vi "Steppers_and_Scanners_control_6_15.vi"(1 "ANC300 address":refnum<visa-resource-name>="COM8") -> (18 "Serial":string="ANC300B-C-2133-4009033")   [LabVIEW 2024]
panel:
  in  "wait time (ms)":u32=300
  out "2: Voltage Reading":dbl format="%#_13g"
  out "1: Voltage Reading":dbl format="%#_13g"
  in  "Set/Read":bool=TRUE
  in  "Stepper 4":bool
  in  "4: number of steps":i32=1
  in  "4: stepping direction":bool=TRUE
  in  "4: AC Voltage":dbl=60.0 min=0.0 format="%.1f"
  in  "4: AC frequency":dbl=300.0 min=0.0 format="%.1f"
  in  "Stepper 3":bool
  in  "3: number of steps":i32=1
  in  "3: stepping direction":bool=TRUE
  in  "3: AC Voltage":dbl=60.0 min=0.0 format="%.1f"
  in  "3: AC frequency":dbl=300.0 min=0.0 format="%.1f"
  in  "2: ms to wait":u32=30
  in  "2: Offset Voltage":dbl min=0.0 format="%.2g"
  in  "1: ms to wait":u32=30
  in  "1: Offset Voltage":dbl min=0.0 format="%.2f"
  # "scanner limits: 150V at 2K. 60V at 300K"
  # "Scanner 1"
  # "Scanner 2"
  # "59"
  # "66"
  # "1. Shouldn't have to change the ms to wait times. \n2. If the piezos aren't moving, it's probably because they need to be exercised first. Best to do that manually\nwith the switches on the board or by moving it here several steps at a time with a high AC voltage. If it doesn't move, you have to rerun the file because it is waiting for it to move and will get stuck there if it isn't moving.\n3. Set 'low temperature' or 'high temperature' limits on the controller manually. You can't do that remotely.  DONT GO ABOVE 60V"
  # "Move Stepper 3 Once"
  # "Move Stepper 4 Once"
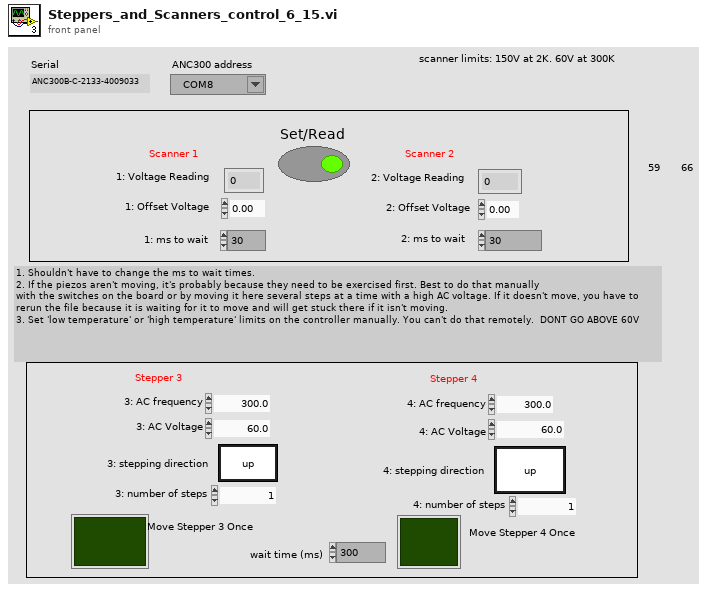
[diagram p1: front panel]
types:
  T1 = cluster{"error ":bool, "error number":i32, "error code":string}
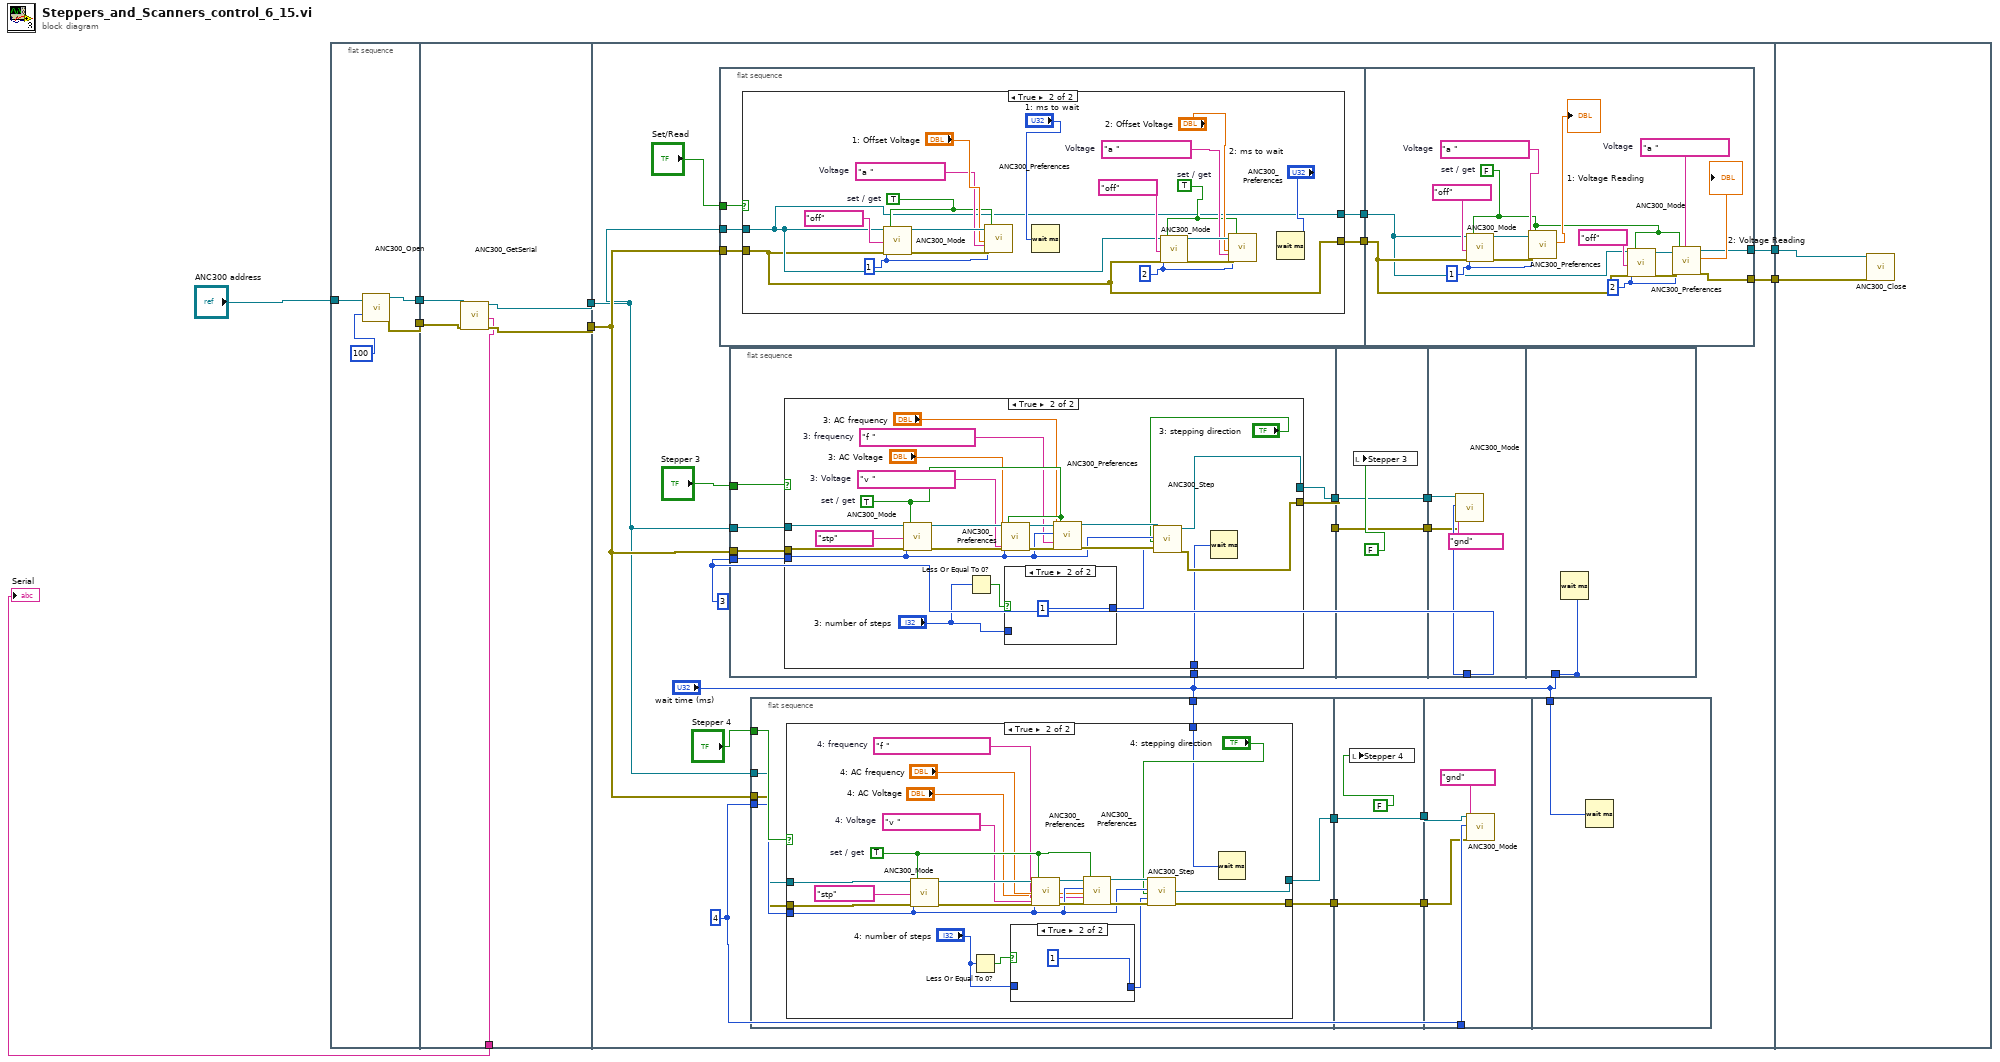
[diagram p0: block diagram]
diagram:
  n1 = flat-sequence {
    tunnel: "ANC300 address" -> [w11]
    tunnel: [w12] -> w8
    tunnel: [w10] -> w7
    tunnel: w8 -> [w17]
    tunnel: w7 -> [w16]
    tunnel: [w15] -> w6
    tunnel: [w14] -> w5
    tunnel: [w13] -> w4
    tunnel: w6 -> [w34]
    tunnel: w5 -> [w35]
    tunnel: [w19] -> w2
    tunnel: [w18] -> w1
    tunnel: w2 -> [w163]
    tunnel: w1 -> [w162]
    frame #0 {
      n2 = call "ANC300_Open.vi"("ANC300 Communication Port In"=w11, "milliseconds to wait"=u32 100 ("millisecond timer value")) -> ("ANC300 Communication Port Out"=w12:refnum<visa-resource-name>, "error out"=w10:T1)  [unwired: 13 in, 3 out]
    }
    frame #1 {
      n3 = call "ANC300_GetSerial.vi"("ANC300 Communication Port In"=w17, "error in"=w16) -> ("ANC300 Communication Port Out"=w15:refnum<visa-resource-name>, "Serial"=w13:string, "error out"=w14:T1)  [unwired: 10 in, 5 out]
    }
    frame #2 {
      w33 = 3
      w36 = 4
      n4 = flat-sequence {
        tunnel: w35 -> [w42]
        tunnel: w34 -> [w41]
        tunnel: "Set/Read" -> [w40]
        tunnel: [w39] -> w26
        tunnel: [w38] -> w25
        tunnel: w26 -> [w68]
        tunnel: w25 -> [w69]
        tunnel: [w64] -> w19
        tunnel: [w63] -> w18
        frame #0 {
          n5 = case shown="True" w40 {
            tunnel: w42 -> [w43 w45]
            tunnel: w41 -> [w44 w46]
            tunnel: [w44 w46] -> w39
            tunnel: [w43 w45] -> w38
            frame False {
            }
            frame True {
              w47 = 2
              w48 = 1
              w49 = TRUE  # set / get
              w52 = "a "  # Voltage
              w56 = TRUE  # set / get
              w59 = "a "  # Voltage
              n6 = call "ANC300_Mode.vi"("ANC300 Communication Port In"=w46, "Axis"=w48, "axis mode in"="off", "error in"=w45, "set / get"=w56) -> ("ANC300 Communication Port Out"=w62:refnum<visa-resource-name>, "error out"=w61:T1)  [unwired: 8 in, 5 out]
              n7 = call "ANC300_Preferences.vi"("ANC300 Communication Port In"=w62, "Axis"=w48, "value in"="1: Offset Voltage", "parameter"=w59, "error in"=w61, "set / get"=w56) -> ()  [unwired: 6 in, 8 out]
              n8 = Wait (ms)(milliseconds to wait="1: ms to wait") -> ()  [unwired: 1 out]
              n9 = call "ANC300_Mode.vi"("ANC300 Communication Port In"=w46, "Axis"=w47, "axis mode in"="off", "error in"=w45, "set / get"=w49) -> ("ANC300 Communication Port Out"=w55:refnum<visa-resource-name>, "error out"=w54:T1)  [unwired: 8 in, 5 out]
              n10 = call "ANC300_Preferences.vi"("ANC300 Communication Port In"=w55, "Axis"=w47, "value in"="2: Offset Voltage", "parameter"=w52, "error in"=w54, "set / get"=w49) -> ()  [unwired: 6 in, 8 out]
              n11 = Wait (ms)(milliseconds to wait="2: ms to wait") -> ()  [unwired: 1 out]
            }
          }
        }
        frame #1 {
          w70 = 2
          w71 = 1
          w73 = "a "  # Voltage
          w65 = FALSE  # set / get
          w77 = "a "  # Voltage
          n12 = call "ANC300_Mode.vi"("ANC300 Communication Port In"=w68, "Axis"=w71, "axis mode in"="off", "error in"=w69, "set / get"=w65) -> ("ANC300 Communication Port Out"=w79:refnum<visa-resource-name>, "error out"=w78:T1)  [unwired: 8 in, 5 out]
          n13 = call "ANC300_Preferences.vi"("ANC300 Communication Port In"=w79, "Axis"=w71, "parameter"=w77, "error in"=w78, "set / get"=w65) -> ("value out"=→"1: Voltage Reading":dbl)  [unwired: 7 in, 7 out]
          n14 = call "ANC300_Mode.vi"("ANC300 Communication Port In"=w68, "Axis"=w70, "axis mode in"="off", "error in"=w69, "set / get"=w65) -> ("ANC300 Communication Port Out"=w75:refnum<visa-resource-name>, "error out"=w74:T1)  [unwired: 8 in, 5 out]
          n15 = call "ANC300_Preferences.vi"("ANC300 Communication Port In"=w75, "Axis"=w70, "parameter"=w73, "error in"=w74, "set / get"=w65) -> ("ANC300 Communication Port Out"=w64:refnum<visa-resource-name>, "value out"=→"2: Voltage Reading":dbl, "error out"=w63:T1)  [unwired: 7 in, 5 out]
        }
      }
      n16 = flat-sequence {
        tunnel: "Stepper 3" -> [w86]
        tunnel: w33 -> [w85]
        tunnel: w34 -> [w84]
        tunnel: w35 -> [w83]
        tunnel: [w82] -> w28
        tunnel: [w81] -> w23
        tunnel: "wait time (ms)" -> [w80]
        tunnel: [w114] -> w29
        tunnel: w28 -> [w114]
        tunnel: [w113] -> w24
        tunnel: w23 -> [w113]
        tunnel: w33 -> [w118]
        tunnel: w29 -> [w117]
        tunnel: w24 -> [w116]
        tunnel: "wait time (ms)" -> [w120]
        tunnel: [w120] -> _
        frame #0 {
          n17 = case shown="True" w86 {
            tunnel: w84 -> [w88 w110]
            tunnel: w85 -> [_ w102]
            tunnel: w83 -> [w87 w107]
            tunnel: [w88 w101] -> w82
            tunnel: [w87 w93] -> w81
            tunnel: w80 -> [_ w92]
            frame False {
            }
            frame True {
              w95 = "v "  # 3: Voltage
              w97 = "f "  # 3: frequency
              w100 = TRUE  # set / get
              n18 = call "ANC300_Mode.vi"("ANC300 Communication Port In"=w110, "Axis"=w102, "axis mode in"="stp", "error in"=w107, "set / get"=w100) -> ("ANC300 Communication Port Out"=w109:refnum<visa-resource-name>, "error out"=w106:T1)  [unwired: 8 in, 5 out]
              n19 = Less Or Equal To 0?(x="3: number of steps") -> (x <= 0?=w90:bool)
              n20 = call "ANC300_Preferences.vi"("ANC300 Communication Port In"=w109, "Axis"=w102, "value in"="3: AC Voltage", "parameter"=w95, "error in"=w106, "set / get"=w100) -> ("ANC300 Communication Port Out"=w104:refnum<visa-resource-name>, "error out"=w103:T1)  [unwired: 6 in, 6 out]
              n21 = case shown="True" w90 {
                tunnel: "3: number of steps" -> [w111 _]
                tunnel: [w111 1] -> w89
                frame False {
                }
                frame True {
                }
              }
              n22 = call "ANC300_Preferences.vi"("ANC300 Communication Port In"=w104, "Axis"=w102, "value in"="3: AC frequency", "parameter"=w97, "error in"=w103, "set / get"=w100) -> ("ANC300 Communication Port Out"=w108:refnum<visa-resource-name>, "error out"=w105:T1)  [unwired: 6 in, 6 out]
              n23 = call "ANC300_Step.vi"("ANC300 Communication Port In"=w108, "Axis"=w102, "stepping direction"="3: stepping direction", "number of steps [0=cont.]"=w89, "error in"=w105) -> ("ANC300 Communication Port Out"=w101:refnum<visa-resource-name>, "error out"=w93:T1)  [unwired: 9 in, 4 out]
              n24 = Wait (ms)(milliseconds to wait=w92) -> ()  [unwired: 1 out]
            }
          }
        }
        frame #1 {
          n25 = local write "Stepper 3"(FALSE) -> ()
        }
        frame #2 {
          n26 = call "ANC300_Mode.vi"("ANC300 Communication Port In"=w117, "Axis"=w118, "axis mode in"="gnd" ("3 Stepper x"), "error in"=w116) -> ()  [unwired: 9 in, 7 out]
        }
        frame #3 {
          n27 = Wait (ms)(milliseconds to wait=w120) -> ()  [unwired: 1 out]
        }
      }
      n28 = flat-sequence {
        tunnel: "Stepper 4" -> [w127]
        tunnel: w36 -> [w126]
        tunnel: w34 -> [w125]
        tunnel: w35 -> [w124]
        tunnel: [w123] -> w30
        tunnel: [w122] -> w21
        tunnel: "wait time (ms)" -> [w121]
        tunnel: [w155] -> w31
        tunnel: w30 -> [w155]
        tunnel: [w154] -> w22
        tunnel: w21 -> [w154]
        tunnel: w36 -> [w159]
        tunnel: w31 -> [w158]
        tunnel: w22 -> [w157]
        tunnel: "wait time (ms)" -> [w161]
        frame #0 {
          n29 = case shown="True" w127 {
            tunnel: w125 -> [w129 w151]
            tunnel: w126 -> [_ w143]
            tunnel: w124 -> [w128 w148]
            tunnel: [w129 w142] -> w123
            tunnel: [w128 w134] -> w122
            tunnel: w121 -> [_ w133]
            frame False {
            }
            frame True {
              w139 = "v "  # 4: Voltage
              w137 = "f "  # 4: frequency
              w141 = TRUE  # set / get
              n30 = call "ANC300_Mode.vi"("ANC300 Communication Port In"=w151, "Axis"=w143, "axis mode in"="stp", "error in"=w148, "set / get"=w141) -> ("ANC300 Communication Port Out"=w150:refnum<visa-resource-name>, "error out"=w147:T1)  [unwired: 8 in, 5 out]
              n31 = Less Or Equal To 0?(x="4: number of steps") -> (x <= 0?=w130:bool)
              n32 = case shown="True" w130 {
                tunnel: "4: number of steps" -> [w152 _]
                tunnel: [w152 1] -> w131
                frame False {
                }
                frame True {
                }
              }
              n33 = call "ANC300_Preferences.vi"("ANC300 Communication Port In"=w150, "Axis"=w143, "value in"="4: AC Voltage", "parameter"=w139, "error in"=w147, "set / get"=w141) -> ("ANC300 Communication Port Out"=w145:refnum<visa-resource-name>, "error out"=w144:T1)  [unwired: 6 in, 6 out]
              n34 = call "ANC300_Preferences.vi"("ANC300 Communication Port In"=w145, "Axis"=w143, "value in"="4: AC frequency", "parameter"=w137, "error in"=w144, "set / get"=w141) -> ("ANC300 Communication Port Out"=w149:refnum<visa-resource-name>, "error out"=w146:T1)  [unwired: 6 in, 6 out]
              n35 = call "ANC300_Step.vi"("ANC300 Communication Port In"=w149, "Axis"=w143, "stepping direction"="4: stepping direction", "number of steps [0=cont.]"=w131, "error in"=w146) -> ("ANC300 Communication Port Out"=w142:refnum<visa-resource-name>, "error out"=w134:T1)  [unwired: 9 in, 4 out]
              n36 = Wait (ms)(milliseconds to wait=w133) -> ()  [unwired: 1 out]
            }
          }
        }
        frame #1 {
          n37 = local write "Stepper 4"(FALSE) -> ()
        }
        frame #2 {
          n38 = call "ANC300_Mode.vi"("ANC300 Communication Port In"=w158, "Axis"=w159, "axis mode in"="gnd" ("3 Stepper x"), "error in"=w157) -> ()  [unwired: 9 in, 7 out]
        }
        frame #3 {
          n39 = Wait (ms)(milliseconds to wait=w161) -> ()  [unwired: 1 out]
        }
      }
    }
    frame #3 {
      n40 = call "ANC300_Close.vi"("ANC300 Communication Port In"=w163, "error in"=w162) -> ()  [unwired: 17 in, 1 out]
    }
  }
  "Serial" <- w4
